vi "输入功能全局.vi"(10 "输入":T1, 11 "选项":enum16{"initialize", "read", "write"}(ring)) -> (3 "输入 2":T1)   [LabVIEW 2017]
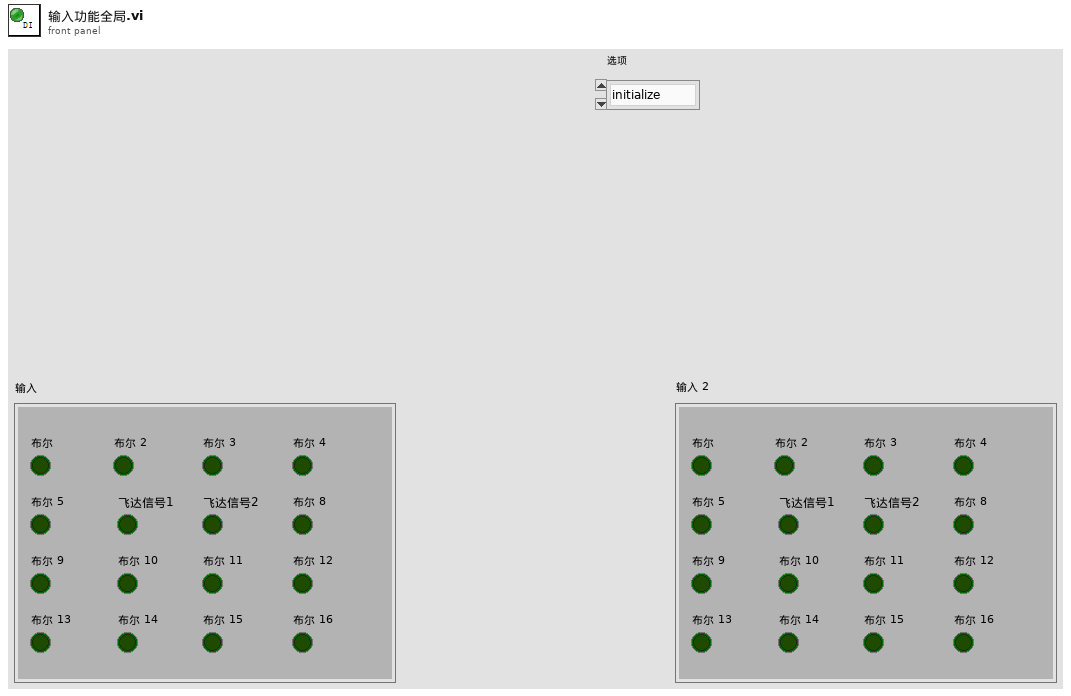
[diagram p1: front panel]
types:
  T1 = typedef "input控件.ctl" = cluster{"布尔":bool, "布尔 2":bool, "布尔 3":bool, "布尔 4":bool, "布尔 5":bool, "飞达信号1":bool, "飞达信号2":bool, "布尔 8":bool, "布尔 9":bool, "布尔 10":bool, "布尔 11":bool, "布尔 12":bool, "布尔 13":bool, "布尔 14":bool, "布尔 15":bool, "布尔 16":bool}
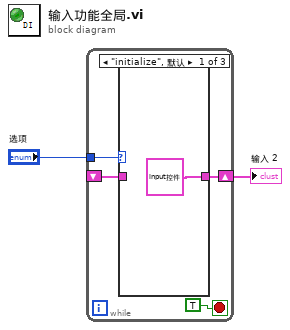
[diagram p0: block diagram]
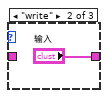
[diagram p2: hidden frame]
diagram:
  n1 = while {
    shift-right: [w5] -> w2
    shift-left: _ -> [w3]
    tunnel: "选项" -> [w4]
    stop <- TRUE stop-if-true
    n2 = case shown="\"initialize\", 默认" w4 {
      tunnel: [T1 {"布尔"=FALSE, "布尔 2"=FALSE, "布尔 3"=FALSE, "布尔 4"=FALSE, "布尔 5"=FALSE, "飞达信号1"=FALSE, "飞达信号2"=FALSE, "布尔 8"=FALSE, "布尔 9"=FALSE, "布尔 10"=FALSE, "布尔 11"=FALSE, "布尔 12"=FALSE, "布尔 13"=FALSE, "布尔 14"=FALSE, "布尔 15"=FALSE, "布尔 16"=FALSE} ("输入") "输入" w9] -> w5
      tunnel: w3 -> [_ _ w9]
      frame "initialize", Default {
      }
      frame "write" {
      }
      frame "read" {
      }
    }
  }
  "输入 2" <- w2
